vi "Set.vi"(8 "error in":errorcluster, 9 "timeout ms (2000)":i32=2000, 10 "SCPI Message":string="ACQ:BUF:SIZE?", 11 "RedPitaya connection in":refnum<k5>) -> (0 "error out":errorcluster, 1 "bytes written":i32, 3 "RedPitaya connection out":refnum<k5>)   [LabVIEW 2010, in "RedPitaya.lvlib"]
uses:
  RedPitaya.lvlib
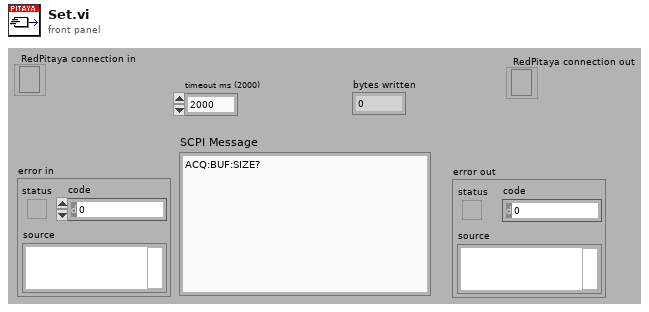
[diagram p1: front panel]
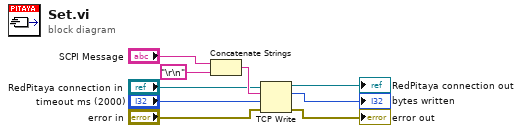
[diagram p0: block diagram]
diagram:
  n1 = Concatenate Strings("SCPI Message", "\r\n") -> (w7:string)
  n2 = TCP Write(connection ID="RedPitaya connection in", data in=w7, error in (no error)="error in", 9:"timeout ms (2000)") -> (connection ID out=→"RedPitaya connection out":refnum<k5>, bytes written=→"bytes written":i32, error out=→"error out":errorcluster)
